vi "test xfer.vi"() -> ()   [LabVIEW 2013, in "DMA.lvclass"]
uses:
  DMA.lvclass
  NOAA Wide/NOAA Wide.lvclass
  DMA.lvclass/DMA.ctl
  Atmospheric/Gas Properties/Gas Properties.lvclass/Gas Properties.ctl
  Accessors/Read Gas Ref.vi
  Accessors/Write Qex.vi
  Accessors/Write Qsh.vi
  Atmospheric/Gas Properties/Accessors/Write P (mb).vi
  Atmospheric/Gas Properties/Accessors/Write T (K).vi
  Conversion Constants.vi
  Atmospheric/Gas Properties/Gas Properties.lvclass
panel:
  out "xfer":dbl[][](array[numeric]) format="%#.2g"
  out "Array":dbl[](array[numeric])
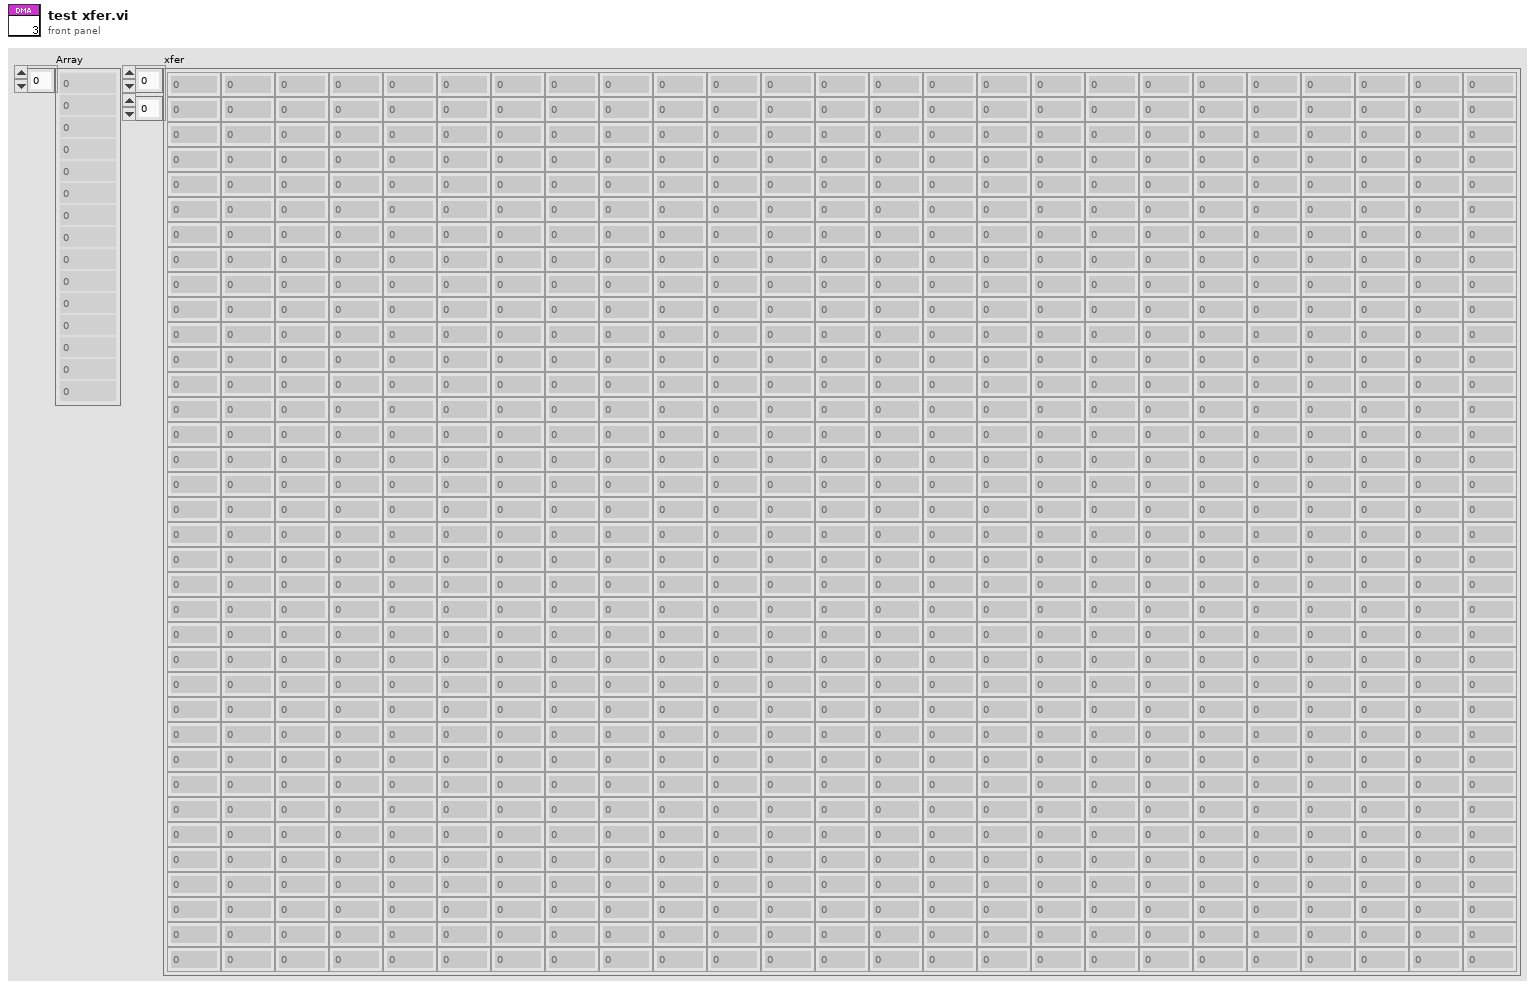
[diagram p1: front panel]
types:
  T1 = cluster{"Vlow":dbl, "Vhigh":dbl, "tscan":i32, "tdwell":i32, "Scan?":bool}
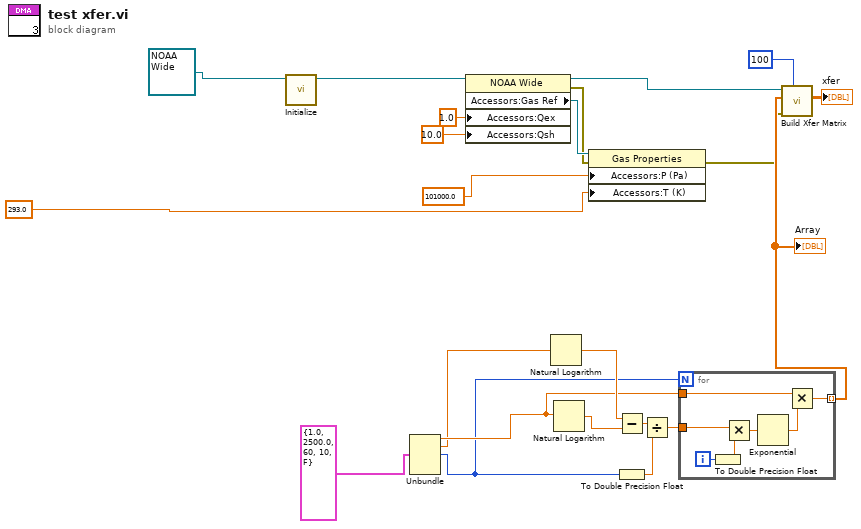
[diagram p0: block diagram]
diagram:
  n1 = call-dynamic "Initialize.vi"("NOAA Wide in"=refnum<class "NOAA Wide.lvclass"> refnum ("NOAA Wide")) -> ("NOAA Wide out"=w7:refnum<class "NOAA Wide.lvclass">)  [unwired: 9 in, 1 out]
  n2 = Unbundle(T1 {"Vlow"=1.0, "Vhigh"=2500.0, "tscan"=60, "tdwell"=10, "Scan?"=FALSE} ("notification")) -> ("Vlow"=w14:dbl, "Vhigh"=w13:dbl, "tscan"=w12:i32)  [unwired: 2 out]
  n3 = property class="NOAA Wide"(reference=w7, "Accessors:Qex"=1.0 ("Qex"), "Accessors:Qsh"=10.0 ("Qsh")) -> (reference out=w20:refnum<class "NOAA Wide.lvclass">, error out=w3:errorcluster, "Accessors:Gas Ref"=w6:refnum<data-value>)  [unwired: 1 in]
  n4 = Natural Logarithm(1:w13) -> (0:w18:dbl)
  n5 = Natural Logarithm(1:w14) -> (0:w19:dbl)
  n6 = property class="Gas Properties"(reference=w6, error in=w3, "Accessors:P (Pa)"=101000.0 ("P (Pa)"), "Accessors:T (K)"=293.0 ("T (K)")) -> (error out=w2:errorcluster)  [unwired: 1 out]
  n7 = Subtract(x=w18, y=w19) -> (x-y=w17:dbl)
  n8 = To Double Precision Float(number=w12) -> (double precision float=w16:dbl)
  n9 = Divide(x=w17, y=w16) -> (x/y=w15:dbl)
  n10 = for {
    N: w12 -> [_]
    tunnel: w15 -> [w28]
    tunnel: w14 -> [w29]
    tunnel: [w23] -> w10 mode=indexing
    i -> [w27]
    n11 = To Double Precision Float(number=w27) -> (double precision float=w26:dbl)
    n12 = Multiply(x=w28, y=w26) -> (x*y=w25:dbl)
    n13 = Exponential(1:w25) -> (0:w24:dbl)
    n14 = Multiply(x=w29, y=w24) -> (x*y=w23:dbl)
  }
  "Array" <- w10
  n15 = call "Build Xfer Matrix.vi"("NumBins"=100, "error in (no error)"=w2, "Voltage"=w10, "DMA in"=w20) -> ("xfer"=→"xfer":dbl[][])  [unwired: 5 in, 2 out]
